vi "Focus Grid Chooser.vi"(10 "SEM Scan Parameters":T2={"X size (um)"=80.0, "Y size (um)"=80.0, "X center (um)"=0.0, "Y center (um)"=0.0, "X size (V)"=3.7333333333333334, "X size auto"=TRUE, "X stig"=[[0.0]], "Y stig"=[[0.0]], "X aln"=[[0.0]], "Y aln"=[[0.0]], "Scan rate (Hz)"=10000000, "Oversampling"=5, "Oversampling auto"=TRUE, "Frame line rampdown ratio"=0.1, "Pixel size (nm)"=8.0, "WD (mm)"=[[3.0]], "X tiles"=1, "Y tiles"=1, "Overlap (um)"=2.0, "Interlaced"=TRUE, "dX (um)"=[0.0], "dY (um)"=[0.0], "Frames"=1} {"dY (um)" format="%.1f"; "dX (um)" format="%.1f"; "Frames" min=1 step=1; "WD (mm)" step=0.001 format="%.4f"; "Y aln" format="%.1f"; "X aln" format="%.1f"; "Y stig" format="%.1f"; "X stig" format="%.1f"; "Overlap (um)" min=0; "Y tiles" min=1; "X tiles" min=1; "X size (um)" format="%.2f"; "Y size (um)" format="%.2f"; "Frame line rampdown ratio" min=0 max=1 step=0.05 format="%.2g"; "X center (um)" step=1 format="%.3f"; "Y center (um)" step=1 format="%.3f"; "X size (V)" format="%_4g"; "Scan rate (Hz)" max=4000000 step=100000 format="%.2e"}, 11 "Focus Index Options":T1={"Keep aspect ratio"=FALSE, "Show Focus Index"=TRUE, "Focus Index primary grid center"=TRUE, "X Grids"=[[1]], "Y Grids"=[[1]], "Primary X index"=[[1]], "Primary Y index"=[[1]]} {"Y Grids" step=2; "X Grids" step=2}) -> (3 "Focus Index Options Out":T1={"Keep aspect ratio"=FALSE, "Show Focus Index"=TRUE, "Focus Index primary grid center"=TRUE, "X Grids"=[[1]], "Y Grids"=[[1]], "Primary X index"=[[1]], "Primary Y index"=[[1]]} {"Y Grids" step=2; "X Grids" step=2})   [LabVIEW 2018]
panel:
  in  "Centered":bool
  out "X Prmry out":u8[][](array[numeric])
  out "Y Prmry out":u8[][](array[numeric])
  out "Tile Y":i32
  out "Tile X":i32
  in  "Tile Grid":bool[][](array[boolean])=[[TRUE, FALSE, FALSE, FALSE, FALSE], [FALSE, FALSE, FALSE, FALSE, FALSE]] caption="Block Face Tile Grid"
  in  "Finished":bool
  out "Y Prmry":u8
  out "X Prmry":u8
  in  "Nx Grids":u8=1 min=1 step=1
  in  "Ny Grids":u8=1 min=1 step=1
  in  "PF Grid":bool[][](array[boolean]) caption="Tile's Primary-Focus Grid"
  # "Grids"
  # "Primary"
  # "Grids"
  # "Primary"
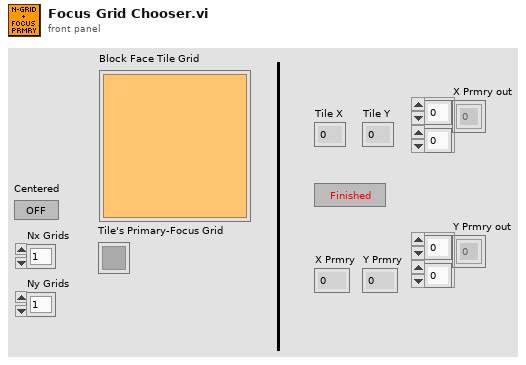
[diagram p1: front panel]
types:
  T1 = cluster{"Keep aspect ratio":bool, "Show Focus Index":bool, "Focus Index primary grid center":bool, "X Grids":u8[][], "Y Grids":u8[][], "Primary X index":u8[][], "Primary Y index":u8[][]}
  T2 = cluster{"X size (um)":sgl, "Y size (um)":sgl, "X center (um)":sgl, "Y center (um)":sgl, "X size (V)":dbl, "X size auto":bool, "X stig":sgl[][], "Y stig":sgl[][], "X aln":sgl[][], "Y aln":sgl[][], "Scan rate (Hz)":u32, "Oversampling":u32, "Oversampling auto":bool, "Frame line rampdown ratio":sgl, "Pixel size (nm)":sgl, "WD (mm)":sgl[][], "X tiles":u8, "Y tiles":u8, "Overlap (um)":sgl, "Interlaced":bool, "dX (um)":sgl[], "dY (um)":sgl[], "Frames":u8}
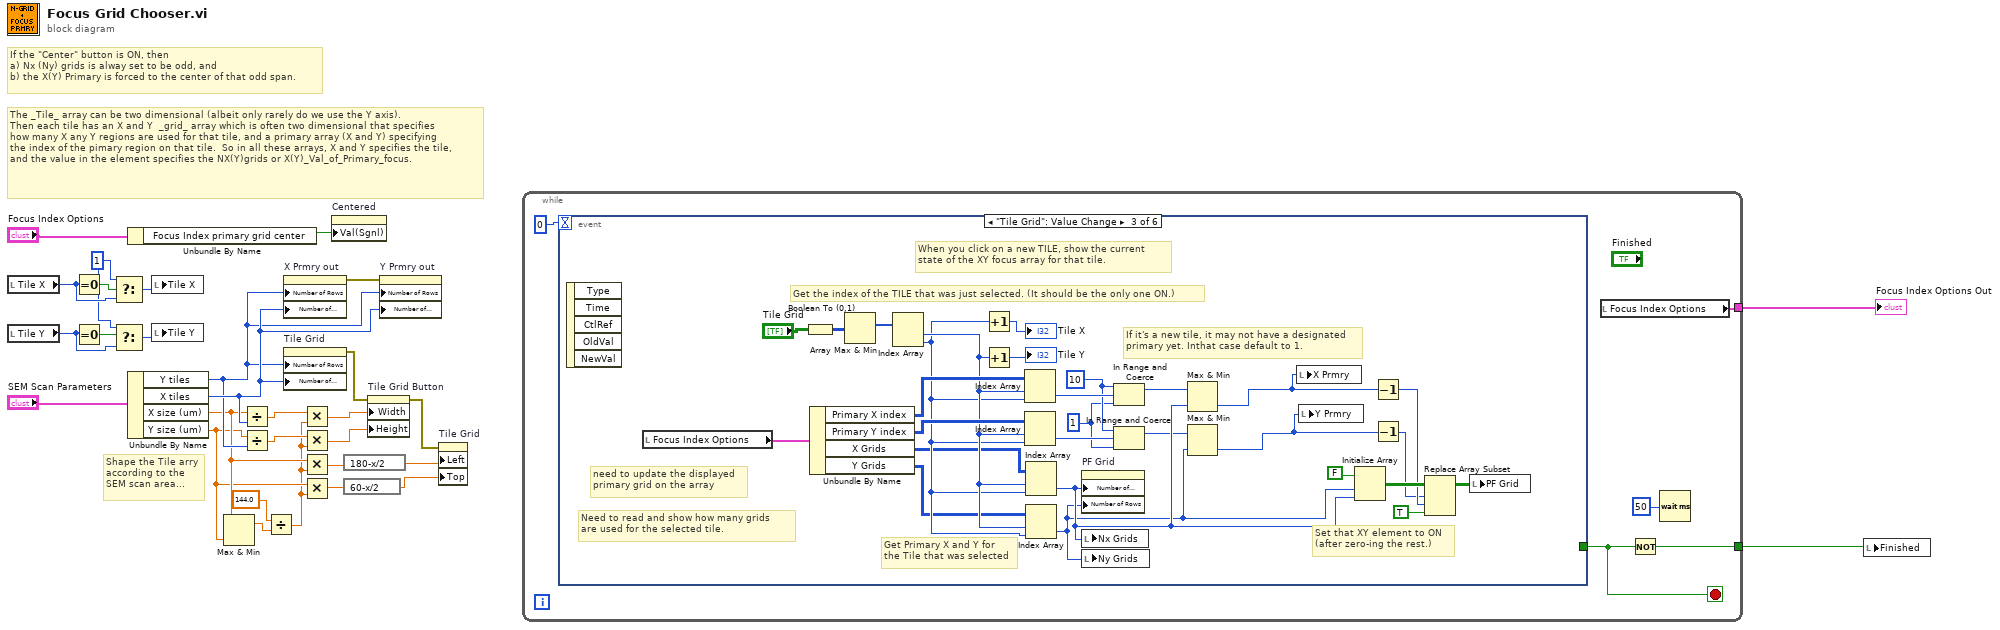
[diagram p0: block diagram]
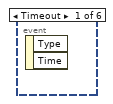
[diagram p2: hidden frame]
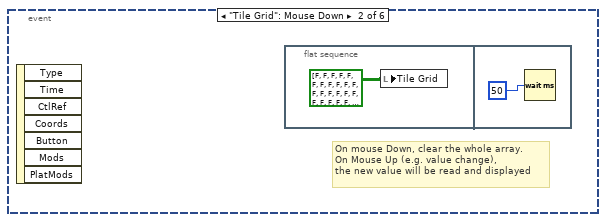
[diagram p3: hidden frame]
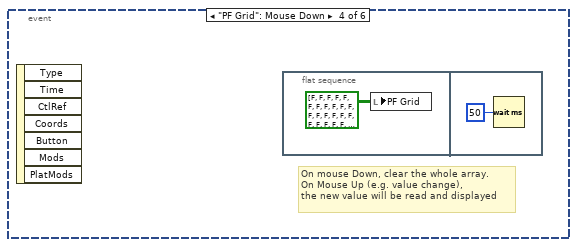
[diagram p4: hidden frame]
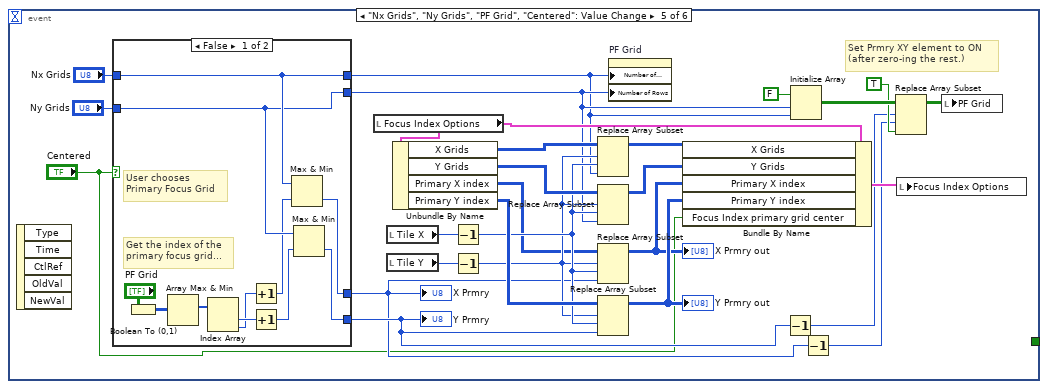
[diagram p5: hidden frame]
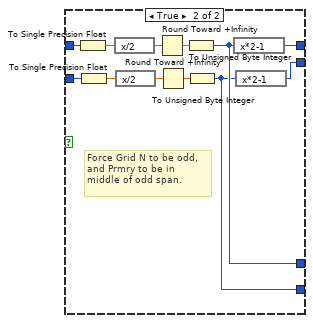
[diagram p6: hidden frame]
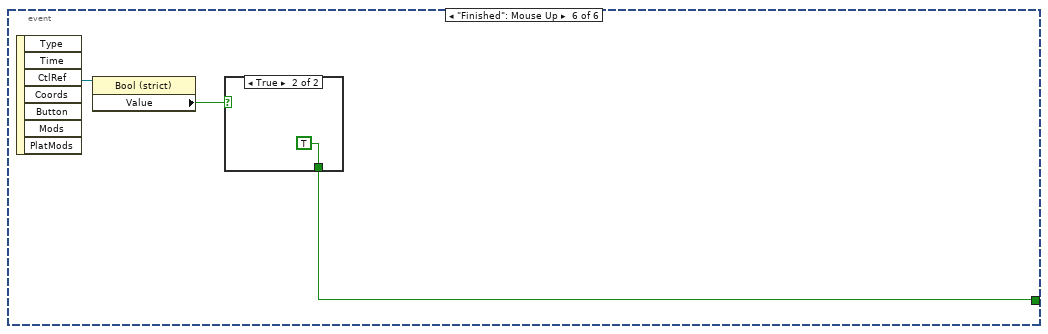
[diagram p7: hidden frame]
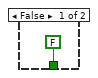
[diagram p8: hidden frame]
diagram:
  w16 = 1 ("t")
  # "Shape the Tile arry\naccording to the\nSEM scan area..."
  # "If the \"Center\" button is ON, then \na) Nx (Ny) grids is alway set to be odd, and \nb) the X(Y) Primary is forced to the center of that odd span."
  # "The _Tile_ array can be two dimensional (albeit only rarely do we use the Y axis).  \nThen each tile has an X and Y  _grid_ array which is often two dimensional that specifies\nhow many X any Y regions are used for that tile, and a primary array (X and Y) specifying\nthe index of the pimary region on that tile.  So in all these arrays, X and Y specifies the tile, \nand the value in the element specifies the NX(Y)grids or X(Y)_Val_of_Primary_focus."
  n1 = local read "Tile X"() -> (w21:i32)
  n2 = local read "Tile Y"() -> (w17:i32)
  n3 = Equal To 0?(x=w21) -> (x = 0?=w22:bool)
  n4 = Equal To 0?(x=w17) -> (x = 0?=w18:bool)
  n5 = Select(t=w16, s=w22, f=w21) -> (s? t:f=w20:i32)
  n6 = Select(t=w16, s=w18, f=w17) -> (s? t:f=w19:i32)
  n7 = Unbundle By Name("Focus Index Options") -> ("Focus Index primary grid center"=w28:bool)
  n8 = Unbundle By Name("SEM Scan Parameters") -> ("Y tiles"=w9:u8, "X tiles"=w10:u8, "X size (um)"=w5:sgl, "Y size (um)"=w4:sgl)
  n9 = local write "Tile X"(w20) -> ()
  n10 = local write "Tile Y"(w19) -> ()
  n11 = Max & Min(x=w5, y=w4) -> (max(x,y)=w1:sgl)  [unwired: 1 out]
  n12 = Divide(x=w5, y=w10) -> (x/y=w11:sgl)
  n13 = Divide(x=w4, y=w9) -> (x/y=w8:sgl)
  n14 = Divide(x=sgl 144.0 ("X size (um)"), y=w1) -> (x/y=w3:sgl)
  n15 = property on="X Prmry out" class="Arr (strict)"("Number of Rows"=w9, "Number of Columns"=w10) -> (error out=w27:errorcluster)  [unwired: 2 in, 1 out]
  n16 = property on="Tile Grid" class="Arr"("Number of Rows"=w9, "Number of Columns"=w10) -> (error out=w30:errorcluster)  [unwired: 2 in, 1 out]
  n17 = Multiply(x=w11, y=w3) -> (x*y=w14:sgl)
  n18 = Multiply(x=w8, y=w3) -> (x*y=w12:sgl)
  n19 = Multiply(x=w5, y=w3) -> (x*y=w7:sgl)
  n20 = Multiply(x=w4, y=w3) -> (x*y=w6:sgl)
  n21 = property on="Centered" class="Bool (strict)"("Val(Sgnl)"=w28) -> ()  [unwired: 2 in, 2 out]
  n22 = expression code="180-x/2"(w7) -> (w15:sgl)
  n23 = expression code="60-x/2"(w6) -> (w13:sgl)
  n24 = property on="Tile Grid Button" class="Bool"(error in=w30, "Width"=w14, "Height"=w12) -> (error out=w29:errorcluster)  [unwired: 1 in, 1 out]
  n25 = property on="Y Prmry out" class="Arr (strict)"(error in=w27, "Number of Rows"=w9, "Number of Columns"=w10) -> ()  [unwired: 1 in, 2 out]
  n26 = property on="Tile Grid" class="Arr"(error in=w29, "Left"=w15, "Top"=w13) -> ()  [unwired: 1 in, 2 out]
  n27 = while {
    tunnel: [w33] -> w24
    tunnel: [w31] -> w23
    stop <- w32 stop-if-true
    n28 = event shown="[2] \"Tile Grid\": Value Change" {
      selector: _ -> [_ _ _ _ _ _]
      dyn-events: _ -> [_ _ _ _ _ _]
      timeout: 0 -> [_ _ _ _ _ _]
      tunnel: [_ _ _ _ _ w118] -> w32
      event Timeout {
        n29 = event-data() -> ()  [unwired: 1 in, 2 out]
      }
      event "Tile Grid": Mouse Down {
        # "On mouse Down, clear the whole array.  \nOn Mouse Up (e.g. value change),\nthe new value will be read and displayed"
        n30 = event-data() -> ()  [unwired: 1 in, 7 out]
        n31 = flat-sequence {
          frame #0 {
            n32 = local write "Tile Grid"(bool[][] [[FALSE, FALSE, FALSE, FALSE, FALSE, FALSE, FALSE, FALSE, FALSE, FALSE, FALSE], [FALSE, FALSE, FALSE, FALSE, FALSE, FALSE, FALSE, FALSE, FALSE, FALSE, FALSE], [FALSE, FALSE, FALSE, FALSE, FALSE, FALSE, FALSE, FALSE, FALSE, FALSE, FALSE], [FALSE, FALSE, FALSE, FALSE, FALSE, FALSE, FALSE, FALSE, FALSE, FALSE, FALSE], [FALSE, FALSE, FALSE, FALSE, FALSE, FALSE, FALSE, FALSE, FALSE, FALSE, FALSE], [FALSE, FALSE, FALSE, FALSE, FALSE, FALSE, FALSE, FALSE, FALSE, FALSE, FALSE], [FALSE, FALSE, FALSE, FALSE, FALSE, FALSE, FALSE, FALSE, FALSE, FALSE, FALSE], [FALSE, FALSE, FALSE, FALSE, FALSE, FALSE, FALSE, FALSE, FALSE, FALSE, FALSE], [FALSE, FALSE, FALSE, FALSE, FALSE, FALSE, FALSE, FALSE, FALSE, FALSE, FALSE], [FALSE, FALSE, FALSE, FALSE, FALSE, FALSE, FALSE, FALSE, FALSE, FALSE, FALSE], [FALSE, FALSE, FALSE, FALSE, FALSE, FALSE, FALSE, FALSE, FALSE, FALSE, FALSE]] ("Tile Primary-Focus Grid")) -> ()
          }
          frame #1 {
            n33 = Wait (ms)(milliseconds to wait=u32 50) -> ()  [unwired: 1 out]
          }
        }
      }
      event "Tile Grid": Value Change {
        w44 = u8 1 ("lower limit")
        w45 = u8 10 ("upper limit")
        # "If it's a new tile, it may not have a designated\nprimary yet. Inthat case default to 1."
        # "Need to read and show how many grids \nare used for the selected tile."
        # "When you click on a new TILE, show the current\nstate of the XY focus array for that tile."
        # "Set that XY element to ON\n(after zero-ing the rest.)"
        # "Get Primary X and Y for\nthe Tile that was selected"
        # "need to update the displayed\nprimary grid on the array"
        # "Get the index of the TILE that was just selected. (It should be the only one ON.)"
        n34 = event-data() -> ()  [unwired: 1 in, 5 out]
        n35 = local read "Focus Index Options"() -> (w60:T1)
        n36 = Boolean To (0,1)(Boolean="Tile Grid") -> (0, 1=w64:i16[][])
        n37 = Unbundle By Name(w60) -> ("Primary X index"=w59:u8[][], "Primary Y index"=w58:u8[][], "X Grids"=w49:u8[][], "Y Grids"=w48:u8[][])
        n38 = Array Max & Min(array=w64) -> (max index (indices)=w63:i32[])  [unwired: 3 out]
        n39 = Index Array(array=w63) -> (element #1=w51:i32, element #2=w50:i32)  [unwired: 2 in]
        n40 = Increment(x=w50) -> (x+1=→"Tile X":i32)
        n41 = Increment(x=w51) -> (x+1=→"Tile Y":i32)
        n42 = Index Array(array=w59, index (row)=w51, index (col)=w50) -> (element=w47:u8)
        n43 = Index Array(array=w58, index (row)=w51, index (col)=w50) -> (element=w46:u8)
        n44 = Index Array(array=w49, index (row)=w51, index (col)=w50) -> (element=w43:u8)
        n45 = Index Array(array=w48, index (row)=w51, index (col)=w50) -> (element=w38:u8)
        n46 = property on="PF Grid" class="Arr"("Number of Columns"=w43, "Number of Rows"=w38) -> ()  [unwired: 2 in, 2 out]
        n47 = local write "Nx Grids"(w43) -> ()
        n48 = local write "Ny Grids"(w38) -> ()
        n49 = In Range and Coerce(upper limit=w45, x=w47, lower limit=w44) -> (coerced(x)=w42:u8)  [unwired: 1 out]
        n50 = In Range and Coerce(upper limit=w45, x=w46, lower limit=w44) -> (coerced(x)=w40:u8)  [unwired: 1 out]
        n51 = Max & Min(x=w42, y=w43) -> (min(x,y)=w41:u8)  [unwired: 1 out]
        n52 = Max & Min(x=w40, y=w38) -> (min(x,y)=w39:u8)  [unwired: 1 out]
        n53 = local write "X Prmry"(w41) -> ()
        n54 = local write "Y Prmry"(w39) -> ()
        n55 = Initialize Array(FALSE, w38, w43) -> (w61:bool[][])
        n56 = Decrement(x=w41) -> (x-1=w53:u8)
        n57 = Decrement(x=w39) -> (x-1=w52:u8)
        n58 = Replace Array Subset(array=w61, new element=TRUE, index (row)=w52, index (col)=w53) -> (w54:bool[][])
        n59 = local write "PF Grid"(w54) -> ()
      }
      event "PF Grid": Mouse Down {
        # "On mouse Down, clear the whole array.  \nOn Mouse Up (e.g. value change),\nthe new value will be read and displayed"
        n60 = event-data() -> ()  [unwired: 1 in, 7 out]
        n61 = flat-sequence {
          frame #0 {
            n62 = local write "PF Grid"(bool[][] [[FALSE, FALSE, FALSE, FALSE, FALSE, FALSE, FALSE, FALSE, FALSE, FALSE, FALSE], [FALSE, FALSE, FALSE, FALSE, FALSE, FALSE, FALSE, FALSE, FALSE, FALSE, FALSE], [FALSE, FALSE, FALSE, FALSE, FALSE, FALSE, FALSE, FALSE, FALSE, FALSE, FALSE], [FALSE, FALSE, FALSE, FALSE, FALSE, FALSE, FALSE, FALSE, FALSE, FALSE, FALSE], [FALSE, FALSE, FALSE, FALSE, FALSE, FALSE, FALSE, FALSE, FALSE, FALSE, FALSE], [FALSE, FALSE, FALSE, FALSE, FALSE, FALSE, FALSE, FALSE, FALSE, FALSE, FALSE], [FALSE, FALSE, FALSE, FALSE, FALSE, FALSE, FALSE, FALSE, FALSE, FALSE, FALSE], [FALSE, FALSE, FALSE, FALSE, FALSE, FALSE, FALSE, FALSE, FALSE, FALSE, FALSE], [FALSE, FALSE, FALSE, FALSE, FALSE, FALSE, FALSE, FALSE, FALSE, FALSE, FALSE], [FALSE, FALSE, FALSE, FALSE, FALSE, FALSE, FALSE, FALSE, FALSE, FALSE, FALSE], [FALSE, FALSE, FALSE, FALSE, FALSE, FALSE, FALSE, FALSE, FALSE, FALSE, FALSE]] ("Tile Primary-Focus Grid")) -> ()
          }
          frame #1 {
            n63 = Wait (ms)(milliseconds to wait=u32 50) -> ()  [unwired: 1 out]
          }
        }
      }
      event "Nx Grids", "Ny Grids", "PF Grid", "Centered": Value Change {
        # "Set Prmry XY element to ON\n(after zero-ing the rest.)"
        n64 = event-data() -> ()  [unwired: 1 in, 5 out]
        n65 = case shown="False" "Centered" {
          tunnel: [w99 w108] -> w76
          tunnel: [w100 w116] -> w75
          tunnel: [w95 w107] -> w70
          tunnel: [w96 w106] -> w72
          tunnel: "Nx Grids" -> [w100 w113]
          tunnel: "Ny Grids" -> [w99 w109]
          frame False {
            # "User chooses \nPrimary Focus Grid"
            # "Get the index of the\nprimary focus grid..."
            n66 = Boolean To (0,1)(Boolean="PF Grid") -> (0, 1=w105:i16[][])
            n67 = Array Max & Min(array=w105) -> (max index (indices)=w104:i32[])  [unwired: 3 out]
            n68 = Index Array(array=w104) -> (element #1=w102:i32, element #2=w101:i32)  [unwired: 2 in]
            n69 = Increment(x=w101) -> (x+1=w98:i32)
            n70 = Increment(x=w102) -> (x+1=w97:i32)
            n71 = Max & Min(x=w100, y=w98) -> (min(x,y)=w95:i32)  [unwired: 1 out]
            n72 = Max & Min(x=w99, y=w97) -> (min(x,y)=w96:i32)  [unwired: 1 out]
          }
          frame True {
            # "Force Grid N to be odd,\nand Prmry to be in\nmiddle of odd span."
            n73 = To Single Precision Float(number=w113) -> (single precision float=w115:sgl)
            n74 = To Single Precision Float(number=w109) -> (single precision float=w111:sgl)
            n75 = expression code="x/2"(w115) -> (w117:sgl)
            n76 = expression code="x/2"(w111) -> (w110:sgl)
            n77 = Round Toward +Infinity(x=w117) -> (ceil(x): smallest int >= x=w114:sgl)
            n78 = Round Toward +Infinity(x=w110) -> (ceil(x): smallest int >= x=w112:sgl)
            n79 = To Unsigned Byte Integer(number=w114) -> (unsigned 8bit integer=w107:u8)
            n80 = To Unsigned Byte Integer(number=w112) -> (unsigned 8bit integer=w106:u8)
            n81 = expression code="x*2-1"(w107) -> (w116:u8)
            n82 = expression code="x*2-1"(w106) -> (w108:u8)
          }
        }
        "X Prmry" <- w70
        "Y Prmry" <- w72
        n83 = local read "Focus Index Options"() -> (w88:T1)
        n84 = local read "Tile X"() -> (w89:i32)
        n85 = local read "Tile Y"() -> (w90:i32)
        n86 = Unbundle By Name(w88) -> ("X Grids"=w93:u8[][], "Y Grids"=w91:u8[][], "Primary X index"=w83:u8[][], "Primary Y index"=w86:u8[][])
        n87 = Decrement(x=w89) -> (x-1=w85:i32)
        n88 = Decrement(x=w90) -> (x-1=w84:i32)
        n89 = Replace Array Subset(array=w93, new element=w75, index (row)=w84, index (col)=w85) -> (w92:u8[][])
        n90 = Replace Array Subset(array=w91, new element=w76, index (row)=w84, index (col)=w85) -> (w87:u8[][])
        n91 = Replace Array Subset(array=w83, new element=w70, index (row)=w84, index (col)=w85) -> (w81:u8[][])
        "X Prmry out" <- w81
        n92 = Replace Array Subset(array=w86, new element=w72, index (row)=w84, index (col)=w85) -> (w82:u8[][])
        "Y Prmry out" <- w82
        n93 = property on="PF Grid" class="Arr"("Number of Columns"=w75, "Number of Rows"=w76) -> ()  [unwired: 2 in, 2 out]
        n94 = Bundle By Name(cluster=w88, "X Grids"=w92, "Y Grids"=w87, "Primary X index"=w81, "Primary Y index"=w82, "Focus Index primary grid center"="Centered") -> (w94:T1)
        n95 = Decrement(x=w72) -> (x-1=w71:i32)
        n96 = Initialize Array(FALSE, w76, w75) -> (w78:bool[][])
        n97 = Decrement(x=w70) -> (x-1=w69:i32)
        n98 = Replace Array Subset(array=w78, new element=TRUE, index (row)=w71, index (col)=w69) -> (w73:bool[][])
        n99 = local write "Focus Index Options"(w94) -> ()
        n100 = local write "PF Grid"(w73) -> ()
      }
      event "Finished": Mouse Up {
        n101 = event-data() -> ("CtlRef"=w120:refnum<vi>)  [unwired: 1 in, 6 out]
        n102 = property class="Bool (strict)"(reference=w120) -> ("Value"=w119:bool)  [unwired: 1 in, 2 out]
        n103 = case shown="True" w119 {
          tunnel: [FALSE ("Finished") TRUE ("Finished")] -> w118
          frame False {
          }
          frame True {
          }
        }
      }
    }
    n104 = local read "Focus Index Options"() -> (w33:T1)
    n105 = Not(x=w32) -> (.not. x?=w31:bool)
    n106 = Wait (ms)(milliseconds to wait=u32 50) -> ()  [unwired: 1 out]
  }
  "Focus Index Options Out" <- w24
  n107 = local write "Finished"(w23) -> ()
